vi "Read Call Chain.vi"(11 "TestManagerMsg.Assertion in":refnum<class "TestManagerMsg.Assertion.lvclass">) -> (2 "Call Chain":string[](array[string]), 3 "TestManagerMsg.Assertion out":refnum<class "TestManagerMsg.Assertion.lvclass">)   [LabVIEW 2020, in "Caraya.lvlib" / "TestManagerMsg.Assertion.lvclass"]
uses:
  TestManagerMsg.Assertion.lvclass
  TestManagerMsg.Assertion.lvclass/TestManagerMsg.Assertion.ctl
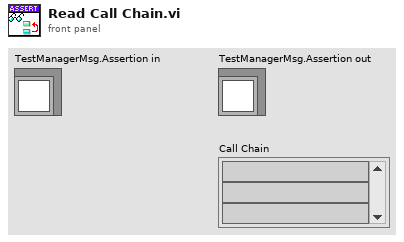
[diagram p1: front panel]
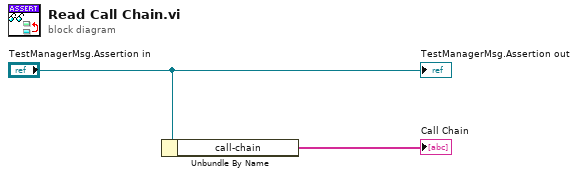
[diagram p0: block diagram]
diagram:
  n1 = Unbundle By Name("TestManagerMsg.Assertion in") -> ("call-chain"=→"Call Chain":string[])
  "TestManagerMsg.Assertion out" <- "TestManagerMsg.Assertion in"
